vi "Determine Teleop State.vi"(11 "Teleop State":T1) -> (2 "Abort":bool, 3 "Teleop State":T1)   [LabVIEW 2017]
uses:
  TypeDefs/ENUM_Overloard States.ctl
  Systems/Overlords/ENUM_Overloard State.ctl
  Systems/Controller/Global Control Outputs.vi
  Systems/Overlords/Overlords.lvlib
  Systems/Controller/Controller.lvlib
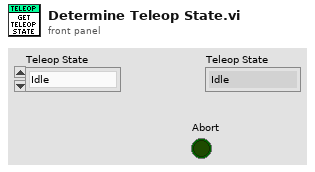
[diagram p1: front panel]
types:
  T1 = typedef "ENUM_Overloard States.ctl" = enum16{"Idle", "Manual", "High Shot", "Low Shot", "Place Gear", "Climb"}
  T2 = typedef "Overlords.lvlib/ENUM_Overloard State.ctl" = enum16{"Idle", "High Shot", "Low Shot", "Place Gear", "Climb"}
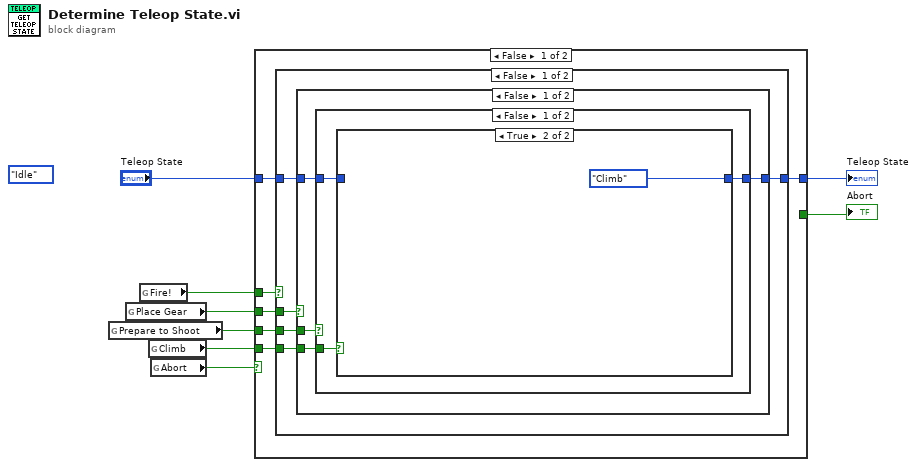
[diagram p0: block diagram]
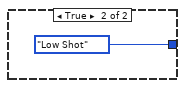
[diagram p3: hidden frame]
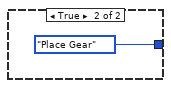
[diagram p4: hidden frame]
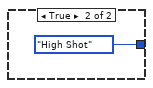
[diagram p5: hidden frame]
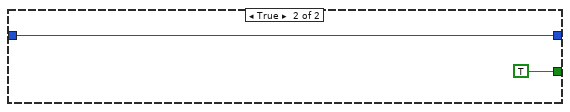
[diagram p6: hidden frame]
diagram:
  (unwired) ENUM_Overloard_State."Idle" ("Teleop State")
  n1 = global read "Global Control Outputs.vi" "Prepare to Shoot"() -> (w2:bool)
  n2 = global read "Global Control Outputs.vi" "Place Gear"() -> (w3:bool)
  n3 = global read "Global Control Outputs.vi" "Fire!"() -> (w4:bool)
  n4 = global read "Global Control Outputs.vi" "Climb"() -> (w1:bool)
  n5 = global read "Global Control Outputs.vi" "Abort"() -> (w8:bool)
  n6 = case shown="False" w8 {
    tunnel: "Teleop State" -> [w14 w33]
    tunnel: [w12 w33] -> w6
    tunnel: [_ TRUE] -> w5
    tunnel: w4 -> [w13 _]
    tunnel: w3 -> [w11 _]
    tunnel: w2 -> [w10 _]
    tunnel: w1 -> [w9 _]
    frame False {
      n7 = case shown="False" w13 {
        tunnel: w14 -> [w19 _]
        tunnel: [w18 ENUM_Overloard_State."High Shot" ("Teleop State")] -> w12
        tunnel: w11 -> [w17 _]
        tunnel: w10 -> [w16 _]
        tunnel: w9 -> [w15 _]
        frame False {
          n8 = case shown="False" w17 {
            tunnel: w19 -> [w23 _]
            tunnel: [w22 ENUM_Overloard_State."Place Gear" ("Teleop State")] -> w18
            tunnel: w16 -> [w21 _]
            tunnel: w15 -> [w20 _]
            frame False {
              n9 = case shown="False" w21 {
                tunnel: w23 -> [w26 _]
                tunnel: [w25 ENUM_Overloard_State."Low Shot" ("Teleop State")] -> w22
                tunnel: w20 -> [w24 _]
                frame False {
                  n10 = case shown="True" w24 {
                    tunnel: w26 -> [w27 _]
                    tunnel: [w27 ENUM_Overloard_State."Climb" ("Teleop State")] -> w25
                    frame False {
                    }
                    frame True {
                    }
                  }
                }
                frame True {
                }
              }
            }
            frame True {
            }
          }
        }
        frame True {
        }
      }
    }
    frame True {
    }
  }
  "Teleop State" <- w6
  "Abort" <- w5
